vi "Start RUS Sweep.vi"(8 "error in (no error)":errorcluster, 11 "RUS Measurement in":refnum<class "RUS Measurement.lvclass">) -> (0 "error out":errorcluster, 3 "RUS Measurement out":refnum<class "RUS Measurement.lvclass">)   [LabVIEW 2015, in "RUS Measurement.lvclass"]
uses:
  RUS Measurement.lvclass
  RUS Parameters.ctl
  Hardware/Spectrum Analyzer Messages/Write Duration Msg/Write Duration Msg.lvclass
  Hardware/Spectrum Analyzer Messages/Write Frequencies Msg/Write Frequencies Msg.lvclass
  Hardware/Spectrum Analyzer Messages/Write Group Name Msg/Write Group Name Msg.lvclass
  Hardware/Spectrum Analyzer Messages/Write Averaging time Msg/Write Averaging time Msg.lvclass
  Mag Lab Root/Mag Lab Root.lvclass/Mag Lab Root.ctl
  RUS Measurement.lvclass/RUS Measurement.ctl
  <vilib>/ActorFramework/Actor/Actor.lvclass/Actor.ctl
  Hardware/Spectrum Analyzer Messages/Write Duration Msg/Write Duration Msg.lvclass/Write Duration Msg.ctl
  Hardware/Spectrum Analyzer Messages/Write Frequencies Msg/Write Frequencies Msg.lvclass/Write Frequencies Msg.ctl
  Hardware/Spectrum Analyzer Messages/Write Group Name Msg/Write Group Name Msg.lvclass/Write Group Name Msg.ctl
  Hardware/Spectrum Analyzer Messages/Write Averaging time Msg/Write Averaging time Msg.lvclass/Write Averaging time Msg.ctl
  Mag Lab Measure Base Messages/Transmit Message Msg/Transmit Message Msg.lvclass/Transmit Message Msg.ctl
  <vilib>/ActorFramework/Message Enqueuer/Message Enqueuer.lvclass/Message Enqueuer.ctl
  Mag Lab Root Messages/Initialize Msg/Initialize Msg.lvclass/Initialize Msg.ctl
  Mag Lab Root/Read Name.vi
  Write Active.vi
  Write Sweep chunk.vi
  Read RUS Instrument.vi
  Mag Lab Root/Read Request time.vi
  <vilib>/ActorFramework/Message Enqueuer/Enqueue.vi
  <vilib>/ActorFramework/Message Priority Queue/Priority Enqueue.vi
  Mag Lab Properties/Mag Lab Parameters.lvclass
  Mag Lab Measure Base Messages/Transmit Message Msg/Transmit Message Msg.lvclass
  Mag Lab Root Messages/Initialize Msg/Initialize Msg.lvclass
  <vilib>/ActorFramework/Actor/Actor.lvclass
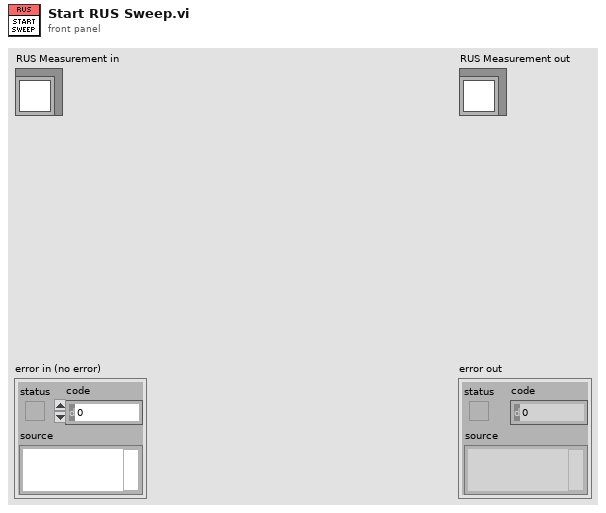
[diagram p1: front panel]
types:
  T1 = typedef "RUS Parameters.ctl" = cluster{"Start frequency":dbl, "End frequency":dbl, "Duration":dbl, "Averaging":dbl, "Find peaks":bool}
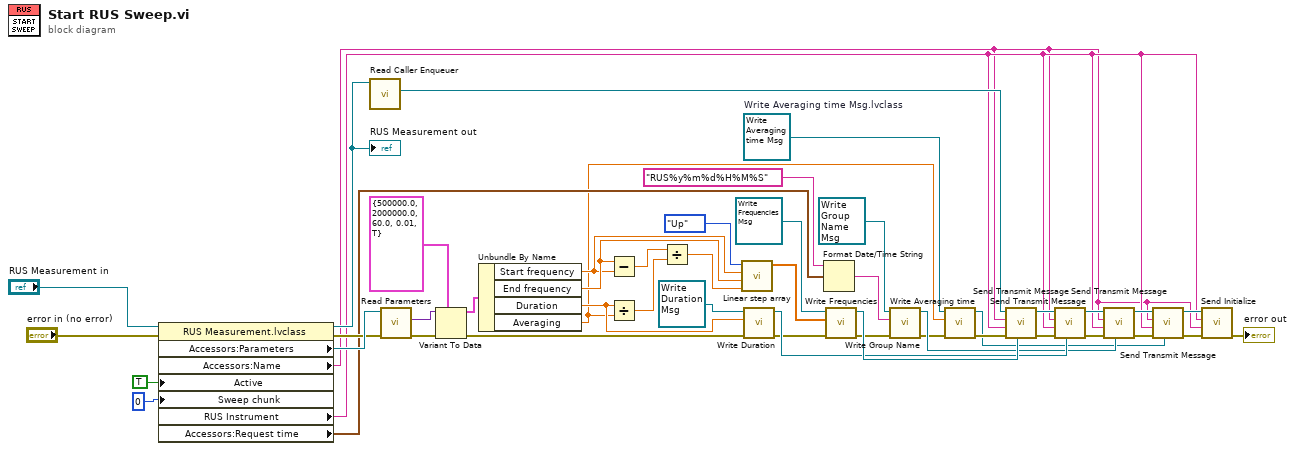
[diagram p0: block diagram]
diagram:
  w4 = refnum<class "Write Averaging time Msg.lvclass"> refnum  # Write Averaging time Msg.lvclass
  n1 = property class="RUS Measurement.lvclass"(reference="RUS Measurement in", error in="error in (no error)", "Active"=TRUE, "Sweep chunk"=0) -> (reference out=w24:refnum<class "RUS Measurement.lvclass">, error out=w21:errorcluster, "Accessors:Parameters"=w22:refnum<class "Mag Lab Parameters.lvclass">, "Accessors:Name"=w1:string, "RUS Instrument"=w2:string, "Accessors:Request time"=w19:timestamp)
  "RUS Measurement out" <- w24
  n2 = call <vilib>:"Read Caller Enqueuer.vi"("Actor"=w24) -> ("Caller Enqueuer"=w27:refnum<class "Message Enqueuer.lvclass">)  [unwired: 10 in]
  n3 = call-dynamic "Read Parameters.vi"("error in (no error)"=w21, "Mag Lab Parameters in"=w22) -> ("error out"=w45:errorcluster, "Parameters"=w44:variant)  [unwired: 7 in, 1 out]
  n4 = Variant To Data(error in=w45, type=T1 {"Start frequency"=500000.0, "End frequency"=2000000.0, "Duration"=60.0, "Averaging"=0.01, "Find peaks"=TRUE} ("Parameters"), Variant=w44) -> (data=w42:T1, error out=w28:errorcluster)
  n5 = Unbundle By Name(w42) -> ("Start frequency"=w40:dbl, "End frequency"=w41:dbl, "Duration"=w33:dbl, "Averaging"=w5:dbl)
  n6 = Subtract(x=w41, y=w40) -> (x-y=w39:dbl)
  n7 = Divide(x=w33, y=w5) -> (x/y=w38:dbl)
  n8 = Divide(x=w39, y=w38) -> (x/y=w37:dbl)
  n9 = call "Linear step array.vi"("Step"=w37, "End"=w41, "Start"=w40, "Mode"=enum16{"Up", "Up-down"}."Up") -> ("Steps"=w35:dbl[])  [unwired: 7 in]
  n10 = call "Write Duration.vi"("error in (no error)"=w28, "Duration"=w33, "Write Duration Msg in"=refnum<class "Write Duration Msg.lvclass"> refnum ("Write Duration Msg.lvclass")) -> ("error out"=w29:errorcluster, "Write Duration Msg out"=w30:refnum<class "Write Duration Msg.lvclass">)  [unwired: 7 in]
  n11 = Format Date/Time String(time format string (%c)="RUS%y%m%d%H%M%S", seconds (now)=w19) -> (date/time string=w17:string)  [unwired: 1 in]
  n12 = call "Write Frequencies.vi"("error in (no error)"=w29, "Frequencies"=w35, "Write Frequencies Msg in"=refnum<class "Write Frequencies Msg.lvclass"> refnum ("Write Frequencies Msg.lvclass")) -> ("error out"=w16:errorcluster, "Write Frequencies Msg out"=w32:refnum<class "Write Frequencies Msg.lvclass">)  [unwired: 7 in]
  n13 = call "Write Group Name.vi"("error in (no error)"=w16, "Group Name"=w17, "Write Group Name Msg in"=refnum<class "Write Group Name Msg.lvclass"> refnum ("Write Group Name Msg.lvclass")) -> ("error out"=w7:errorcluster, "Write Group Name Msg out"=w13:refnum<class "Write Group Name Msg.lvclass">)  [unwired: 7 in]
  n14 = call "Write Averaging time.vi"("error in (no error)"=w7, "Averaging time"=w5, "Write Averaging time Msg in"=w4) -> ("error out"=w6:errorcluster, "Write Averaging time Msg out"=w3:refnum<class "Write Averaging time Msg.lvclass">)  [unwired: 7 in]
  n15 = call "Send Transmit Message.vi"("Message"=w32, "error in (no error)"=w6, "Requestee"=w2, "Requestor"=w1, "Message Enqueuer"=w27) -> ("error out"=w31:errorcluster, "Message Enqueuer out"=w25:refnum<class "Message Enqueuer.lvclass">)  [unwired: 5 in]
  n16 = call "Send Transmit Message.vi"("Message"=w30, "error in (no error)"=w31, "Requestee"=w2, "Requestor"=w1, "Message Enqueuer"=w25) -> ("error out"=w15:errorcluster, "Message Enqueuer out"=w14:refnum<class "Message Enqueuer.lvclass">)  [unwired: 5 in]
  n17 = call "Send Transmit Message.vi"("Message"=w13, "error in (no error)"=w15, "Requestee"=w2, "Requestor"=w1, "Message Enqueuer"=w14) -> ("error out"=w11:errorcluster, "Message Enqueuer out"=w10:refnum<class "Message Enqueuer.lvclass">)  [unwired: 5 in]
  n18 = call "Send Transmit Message.vi"("Message"=w3, "error in (no error)"=w11, "Requestee"=w2, "Requestor"=w1, "Message Enqueuer"=w10) -> ("error out"=w9:errorcluster, "Message Enqueuer out"=w8:refnum<class "Message Enqueuer.lvclass">)  [unwired: 5 in]
  n19 = call "Send Initialize.vi"("error in (no error)"=w9, "Requestor"=w1, "Requestee"=w2, "Message Enqueuer"=w8) -> ("error out"=→"error out":errorcluster)  [unwired: 6 in, 1 out]
